vi "SeCrTs-RPM_Module_A.vi"(7 "Data FIFO Ref":T1, 8 "error in (no error)":errorcluster, 11 "TCP Network Connection in":refnum<k5>) -> (0 "error out":errorcluster, 3 "TCP Network Connection out":refnum<k5>)   [LabVIEW 2022 SP3]
uses:
  RT Controls/ATF Storage-FGV Read write.ctl
  RT Controls/ATF Storage-Data FIFO.ctl
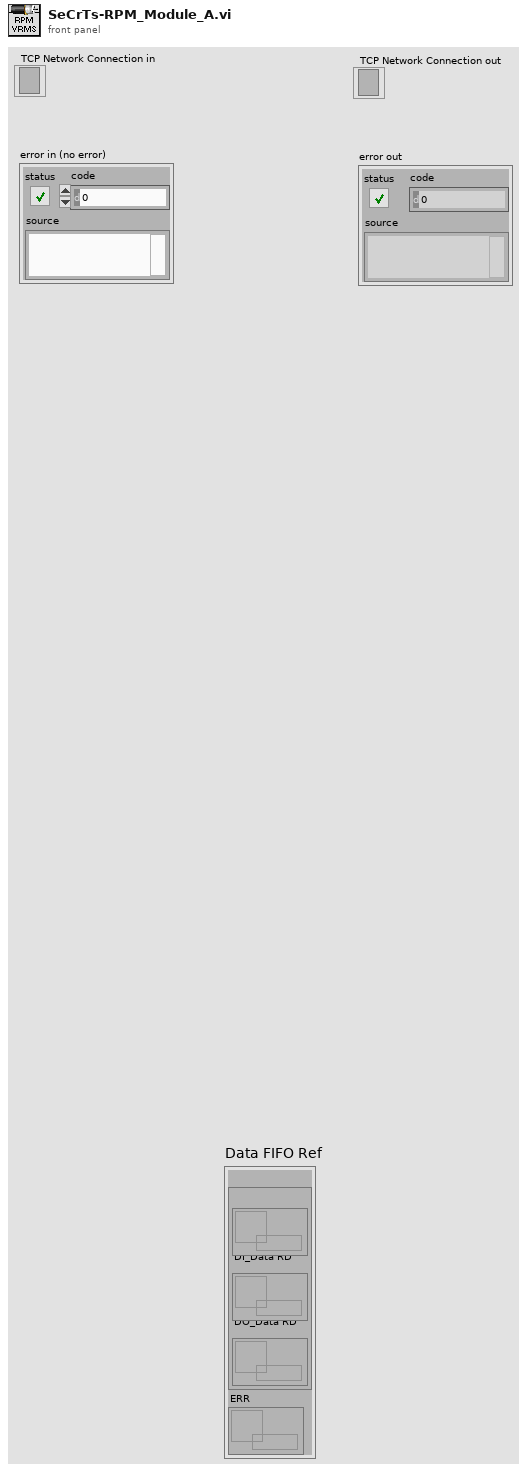
[diagram p1: front panel]
types:
  T1 = typedef "ATF Storage-Data FIFO.ctl" = cluster{"RD":cluster{"AI_V_Data RD":refnum<queue>, "DI_Data RD":refnum<queue>, "DO_Data RD":refnum<queue>}, "ERR":refnum<queue>}
  T2 = enum16{"Standard", "Buffered", "CRLF", "Immediate"}
  T3 = typedef "ATF Storage-FGV Read write.ctl" = enum16{"Write", "Read"}
  T4 = cluster{"En_Drive_A":bool, "En_Drive_L":bool, "Exit_Drive_A":bool, "Exit_Drive_L":bool}
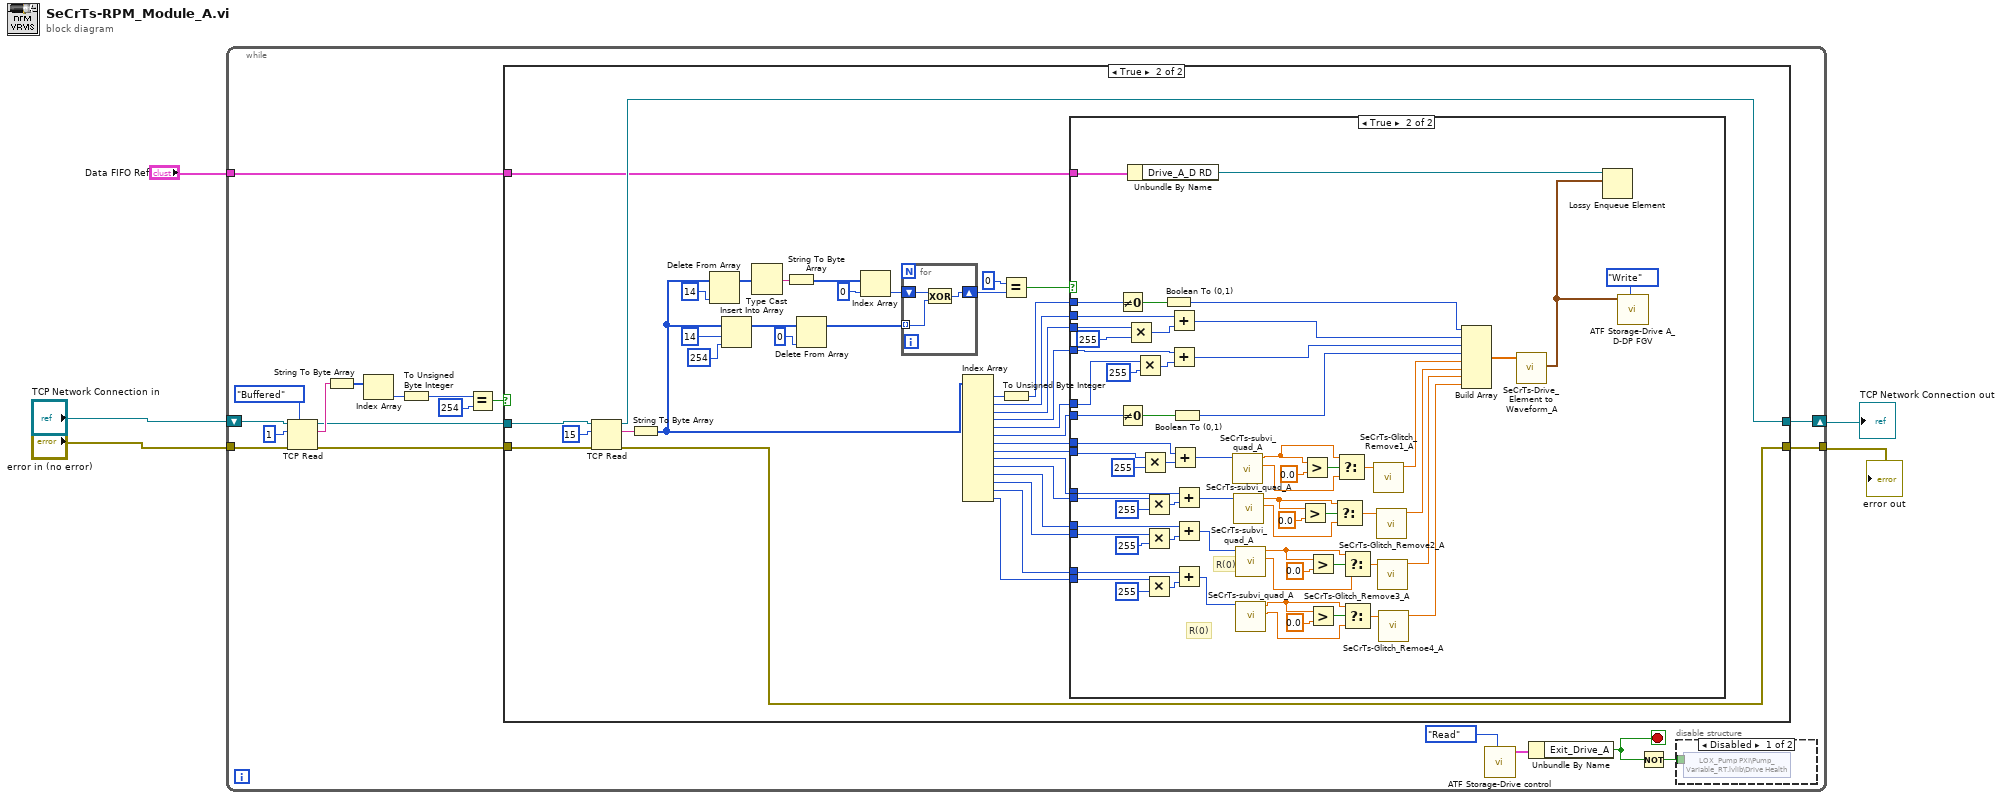
[diagram p0: block diagram]
diagram:
  n1 = while {
    tunnel: "error in (no error)" -> [w23]
    shift-right: [w12] -> w5
    shift-left: "TCP Network Connection in" -> [w24]
    tunnel: [w13] -> w4
    tunnel: "Data FIFO Ref" -> [w6]
    stop <- w7 stop-if-true
    n2 = TCP Read(connection ID=w24, bytes to read=1, error in (no error)=w23, 7:T2."Buffered" ("mode (standard)")) -> (connection ID out=w16:refnum<k5>, data out=w22:string, error out=w15:errorcluster)  [unwired: 1 in]
    n3 = String To Byte Array(string=w22) -> (unsigned byte array=w21:u8[])
    n4 = Index Array(array=w21) -> (element=w20:u8)  [unwired: 1 in]
    n5 = To Unsigned Byte Integer(number=w20) -> (unsigned 8bit integer=w19:u8)
    n6 = Equal?(x=w19, y=u8 254) -> (x = y?=w17:bool)
    n7 = case shown="True" w17 {
      tunnel: w16 -> [w27 w64]
      tunnel: w15 -> [w26 w63]
      tunnel: [w27 w53] -> w12
      tunnel: [w26 w38] -> w13
      tunnel: w6 -> [_ w28]
      frame False {
      }
      frame True {
        n8 = TCP Read(connection ID=w64, bytes to read=15, error in (no error)=w63) -> (connection ID out=w53:refnum<k5>, data out=w61:string, error out=w38:errorcluster)  [unwired: 2 in]
        n9 = String To Byte Array(string=w61) -> (unsigned byte array=w46:u8[])
        n10 = Delete From Array(array=w46, index=14) -> (array with subset deleted=w59:u8[])  [unwired: 1 in, 1 out]
        n11 = Insert Into Array(array=w46, index=14, new element=u8 254 ("new element/subarray")) -> (w52:u8[])
        n12 = Type Cast(x=w59) -> (*(type *) &x=w58:string)  [unwired: 1 in]
        n13 = String To Byte Array(string=w58) -> (unsigned byte array=w57:u8[])
        n14 = Delete From Array(array=w52, index=0) -> (array with subset deleted=w49:u8[])  [unwired: 1 in, 1 out]
        n15 = Index Array(array=w57, index=0) -> (element=w50:u8)
        n16 = for {
          shift-right: [w131] -> w48
          shift-left: w50 -> [w132]
          tunnel: w49 -> [w130] mode=indexing
          n17 = Exclusive Or(1:w130, 2:w132) -> (0:w131:u8)
        }
        n18 = Index Array(array=w46) -> (element #1=w45:u8, element #2=w43:u8, element #3=w42:u8, element #4=w41:u8, element #5=w40:u8, element #6=w39:u8, element #7=w36:u8, element #8=w35:u8, element #9=w34:u8, element #10=w33:u8, element #11=w32:u8, element #12=w31:u8, element #13=w30:u8, element #14=w29:u8)  [unwired: 14 in]
        n19 = Equal?(x=u8 0, y=w48) -> (x = y?=w47:bool)
        n20 = To Unsigned Byte Integer(number=w45) -> (unsigned 8bit integer=w44:u8)
        n21 = case shown="True" w47 {
          tunnel: w44 -> [_ w129]
          tunnel: w43 -> [_ w97]
          tunnel: w42 -> [_ w96]
          tunnel: w41 -> [_ w95]
          tunnel: w40 -> [_ w94]
          tunnel: w39 -> [_ w125]
          tunnel: w36 -> [_ w116]
          tunnel: w35 -> [_ w115]
          tunnel: w34 -> [_ w114]
          tunnel: w33 -> [_ w113]
          tunnel: w32 -> [_ w112]
          tunnel: w31 -> [_ w111]
          tunnel: w30 -> [_ w110]
          tunnel: w29 -> [_ w109]
          tunnel: w28 -> [_ w68]
          frame False {
          }
          frame True {
            # "R(0)"
            # "R(0)"
            n22 = Not Equal To 0?(x=w129) -> (x != 0?=w100:bool)
            n23 = Not Equal To 0?(x=w125) -> (x != 0?=w99:bool)
            n24 = Multiply(x=w96, y=u32 255) -> (x*y=w98:u32)
            n25 = Unbundle By Name(w68) -> ("Drive_A_D RD"=w67:refnum<queue>)
            n26 = Multiply(x=w94, y=u32 255) -> (x*y=w126:u32)
            n27 = Multiply(x=w115, y=u32 255) -> (x*y=w117:u32)
            n28 = Multiply(x=w113, y=u32 255) -> (x*y=w120:u32)
            n29 = Multiply(x=w111, y=u32 255) -> (x*y=w121:u32)
            n30 = Multiply(x=w109, y=u32 255) -> (x*y=w124:u32)
            n31 = Boolean To (0,1)(Boolean=w100) -> (0, 1=w93:i16)
            n32 = Add(x=w97, y=w98) -> (x+y=w92:u32)
            n33 = Add(x=w95, y=w126) -> (x+y=w91:u32)
            n34 = Add(x=w116, y=w117) -> (x+y=w89:u32)
            n35 = Boolean To (0,1)(Boolean=w99) -> (0, 1=w90:i16)
            n36 = Add(x=w114, y=w120) -> (x+y=w86:u32)
            n37 = Add(x=w112, y=w121) -> (x+y=w83:u32)
            n38 = Add(x=w110, y=w124) -> (x+y=w80:u32)
            n39 = call "SeCrTs-subvi_quad_A.vi"("input variable"=w89) -> ("output variable 2"=w87:dbl, "output variable"=w88:dbl)  [unwired: 8 in]
            n40 = call "SeCrTs-subvi_quad_A.vi"("input variable"=w86) -> ("output variable 2"=w84:dbl, "output variable"=w85:dbl)  [unwired: 8 in]
            n41 = call "SeCrTs-subvi_quad_A.vi"("input variable"=w83) -> ("output variable 2"=w81:dbl, "output variable"=w82:dbl)  [unwired: 8 in]
            n42 = call "SeCrTs-subvi_quad_A.vi"("input variable"=w80) -> ("output variable 2"=w78:dbl, "output variable"=w79:dbl)  [unwired: 8 in]
            n43 = Greater?(x=w85, y=0.0) -> (0:w103:bool)
            n44 = Greater?(x=w88, y=0.0) -> (0:w101:bool)
            n45 = Greater?(x=w82, y=0.0) -> (0:w105:bool)
            n46 = Greater?(x=w79, y=0.0) -> (0:w107:bool)
            n47 = Select(t=w85, s=w103, f=w84) -> (s? t:f=w71:dbl)
            n48 = Select(t=w88, s=w101, f=w87) -> (s? t:f=w77:dbl)
            n49 = Select(t=w82, s=w105, f=w81) -> (s? t:f=w73:dbl)
            n50 = Select(t=w79, s=w107, f=w78) -> (s? t:f=w75:dbl)
            n51 = call "SeCrTs-Glitch_Remove1_A.vi"("Input"=w77) -> ("Output"=w76:dbl)  [unwired: 10 in]
            n52 = call "SeCrTs-Glitch_Remove2_A.vi"("Input"=w71) -> ("Output"=w70:dbl)  [unwired: 10 in]
            n53 = call "SeCrTs-Glitch_Remove3_A.vi"("Input"=w73) -> ("Output"=w72:dbl)  [unwired: 10 in]
            n54 = call "SeCrTs-Glitch_Remoe4_A.vi"("Input"=w75) -> ("Output"=w74:dbl)  [unwired: 10 in]
            n55 = Build Array(w93, w92, w91, w90, w76, w70, w72, w74) -> (w69:dbl[])
            n56 = call "SeCrTs-Drive_Element to Waveform_A.vi"("Array input"=w69) -> ("RPM out"=w66:waveform(dbl)[])  [unwired: 10 in]
            n57 = Lossy Enqueue Element(queue=w67, element=w66) -> ()  [unwired: 1 in, 4 out]
            n58 = call "ATF Storage-Drive A_D-DP FGV.vi"("Write/Read"=ATF_Storage-FGV_Read_write."Write", "Drive A_D"=w66) -> ()  [unwired: 8 in, 2 out]
          }
        }
      }
    }
    n59 = call "ATF Storage-Drive control.vi"("Action"=enum16{"Init", "Write", "Read"}."Read") -> ("Loop Control Out"=w8:T4)  [unwired: 9 in, 1 out]
    n60 = Unbundle By Name(w8) -> ("Exit_Drive_A"=w7:bool)
    n61 = Not(x=w7) -> (.not. x?=w10:bool)
    n62 = disable-structure shown="Disabled" {
      disable-tunnel: w10 -> [w25 _]
      frame Disabled {
        n63 = shared-variable "LOX_Pump PXI\\Pump_Variable_RT.lvlib\\Drive Health"(w25) -> ()  [unwired: 1 in, 1 out]
      }
      frame Enabled {
      }
    }
  }
  "TCP Network Connection out" <- w5
  "error out" <- w4
